vi "Test Speichern.vi"() -> ()   [LabVIEW 2020, in "AK-Schnittstelle.lvlib"]
uses:
  AK-Schnittstelle.lvlib
panel:
  out "Recipe Teil":string[][](array[string])
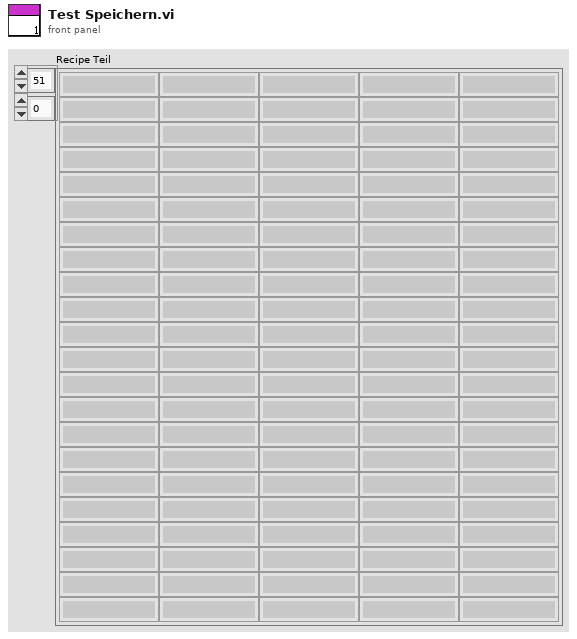
[diagram p1: front panel]
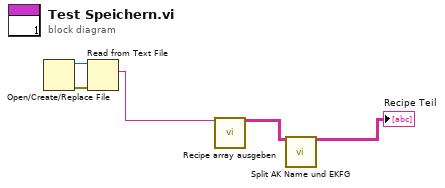
[diagram p0: block diagram]
diagram:
  n1 = Open/Create/Replace File() -> (refnum out=w5:refnum<file>, error out=w4:errorcluster)  [unwired: 6 in, 1 out]
  n2 = Read from Text File(file (use dialog)=w5, error in=w4) -> (text=w3:string)  [unwired: 2 in, 3 out]
  n3 = call "Recipe array ausgeben.vi"("Komplette Datei"=w3) -> ("Recipe Teil"=w2:string[][])  [unwired: 11 in, 3 out]
  n4 = call "Split AK Name und EKFG.vi"("Recipe Teil"=w2) -> ("AK Name"=→"Recipe Teil":string[][])  [unwired: 10 in, 4 out]
